vi "Save.vi"(8 "error in (no error)":errorcluster, 11 "Controller in":refnum<class "Controller.lvclass">) -> (0 "error out":errorcluster, 3 "Controller out":refnum<class "Controller.lvclass">)   [LabVIEW 2013, in "SET Project Editor.lvlib" / "Controller.lvclass"]
uses:
  Controller.lvclass
  Controller.lvclass/Controller.ctl
  SET Project Data/Project Data Class/Project Data.lvclass
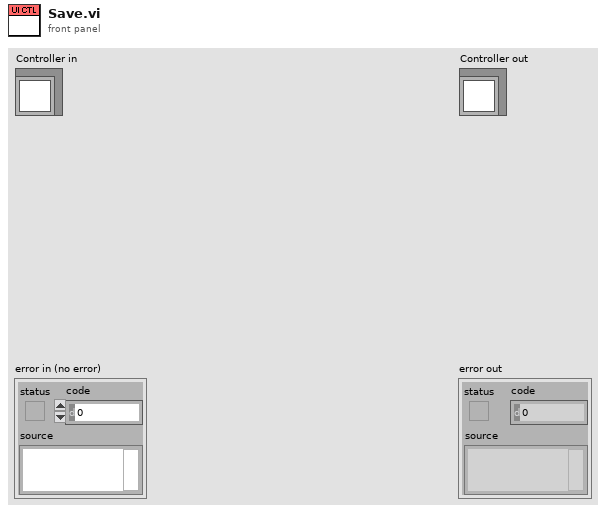
[diagram p1: front panel]
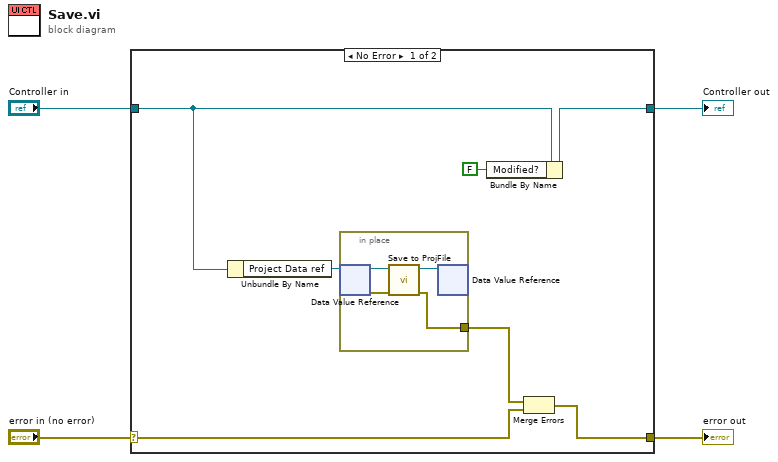
[diagram p0: block diagram]
diagram:
  n1 = case shown="No Error" "error in (no error)" {
    selector: "error in (no error)" -> [w7 w17]
    tunnel: [w6 w17] -> w3
    tunnel: [w5 w16] -> w1
    tunnel: "Controller in" -> [w10 w16]
    frame No Error {
      n2 = Unbundle By Name(w10) -> ("Project Data ref"=w9:refnum<data-value>)
      n3 = in-place {
        in-place-border: [w12] -> w8
        n4 = in-place-dvr #1(w9) -> (w15:refnum<class "Project Data.lvclass">, w13:errorcluster)
        n5 = call "Save to ProjFile.vi"("error in (no error)"=w13, "LanguageData in"=w15) -> ("error out"=w12:errorcluster, "LanguageData out"=w14:refnum<class "Project Data.lvclass">)  [unwired: 8 in]
        n6 = in-place-dvr #1(w14) -> ()  [unwired: 2 out]
      }
      n7 = Bundle By Name(cluster=w10, "Modified?"=FALSE) -> (w5:refnum<class "Controller.lvclass">)
      n8 = Merge Errors(w8, w7) -> (w6:errorcluster)
    }
    frame Error {
    }
  }
  "error out" <- w3
  "Controller out" <- w1
